vi "ProjetoB_59939_60461.vi"() -> ()   [LabVIEW 2024]
uses:
  <vilib>/Instr/_visa.llb/VISA Configure Serial Port (Instr).vi
  <vilib>/Analysis/NI_AALBase.lvlib
panel:
  in  "Help Button":bool
  out "Desvio Padrão Alto":bool
  in  "Limiar Desvio Padrão":dbl
  out "Desvio Padrão":dbl
  out "Frequência":dbl(graph)
  out "Array":dbl[](array[numeric])
  in  "Array - Numeric":dbl[](array[numeric])
  out "Sinal":u8(graph)
  in  "Ignição":bool
  in  "Modo\nAutomático":bool
  in  "Aumentar Frequência\n          Taxa Alta":bool
  in  "Aumentar Frequência\n         Taxa Baixa":bool
  in  "Reduzir \nFrequência":bool
  out "Sem onda há 10s":bool
  out "0.3 < Frequência < 0.6":bool
  in  "Iniciar/Parar \n  Aquisição":bool
  out "Frequência < 0.3":bool
  out "Frequência > 3":bool
  out "Deteção de Onda":bool
  in  "Limiar superior de Deteção":dbl=200.0
  out "Limiar inferior de Deteção":dbl=120.0
  out "Frequência":dbl
  in  "Taxa de Amostragem":u16(ring)=1 items=["25 S/s", "50 S/s", "100 S/s", "200 S/s"]
  in  "Gravar":bool
  out "Último Valor":dbl
  out "Error Out":errorcluster
  in  "stop":bool
  in  "Error In (no error)":errorcluster
  in  "Nome da Fonte VISA":refnum<visa-resource-name>="COM4"
  # "Monitorização de Plasma"
  # "Instrumentação Digital"
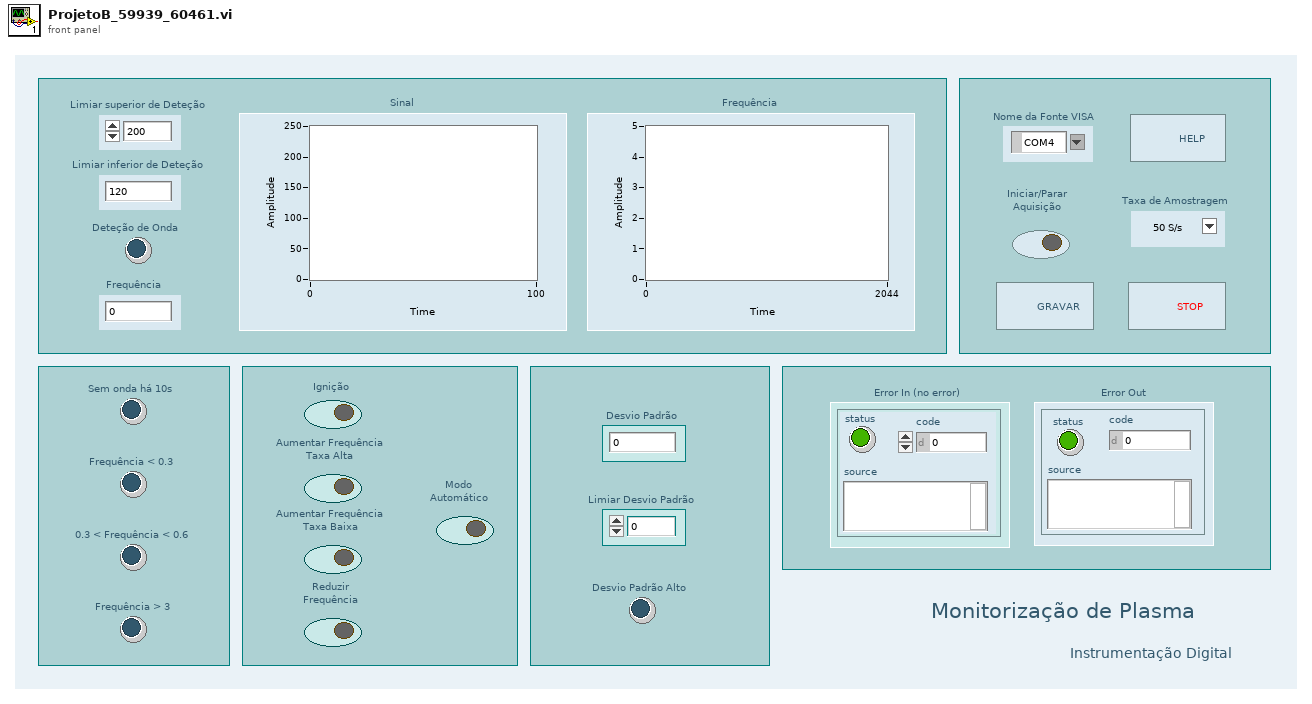
[diagram p1: front panel]
types:
  T1 = enum16{"open", "replace", "create", "open or create", "replace or create", "replace or create with confirmation"}
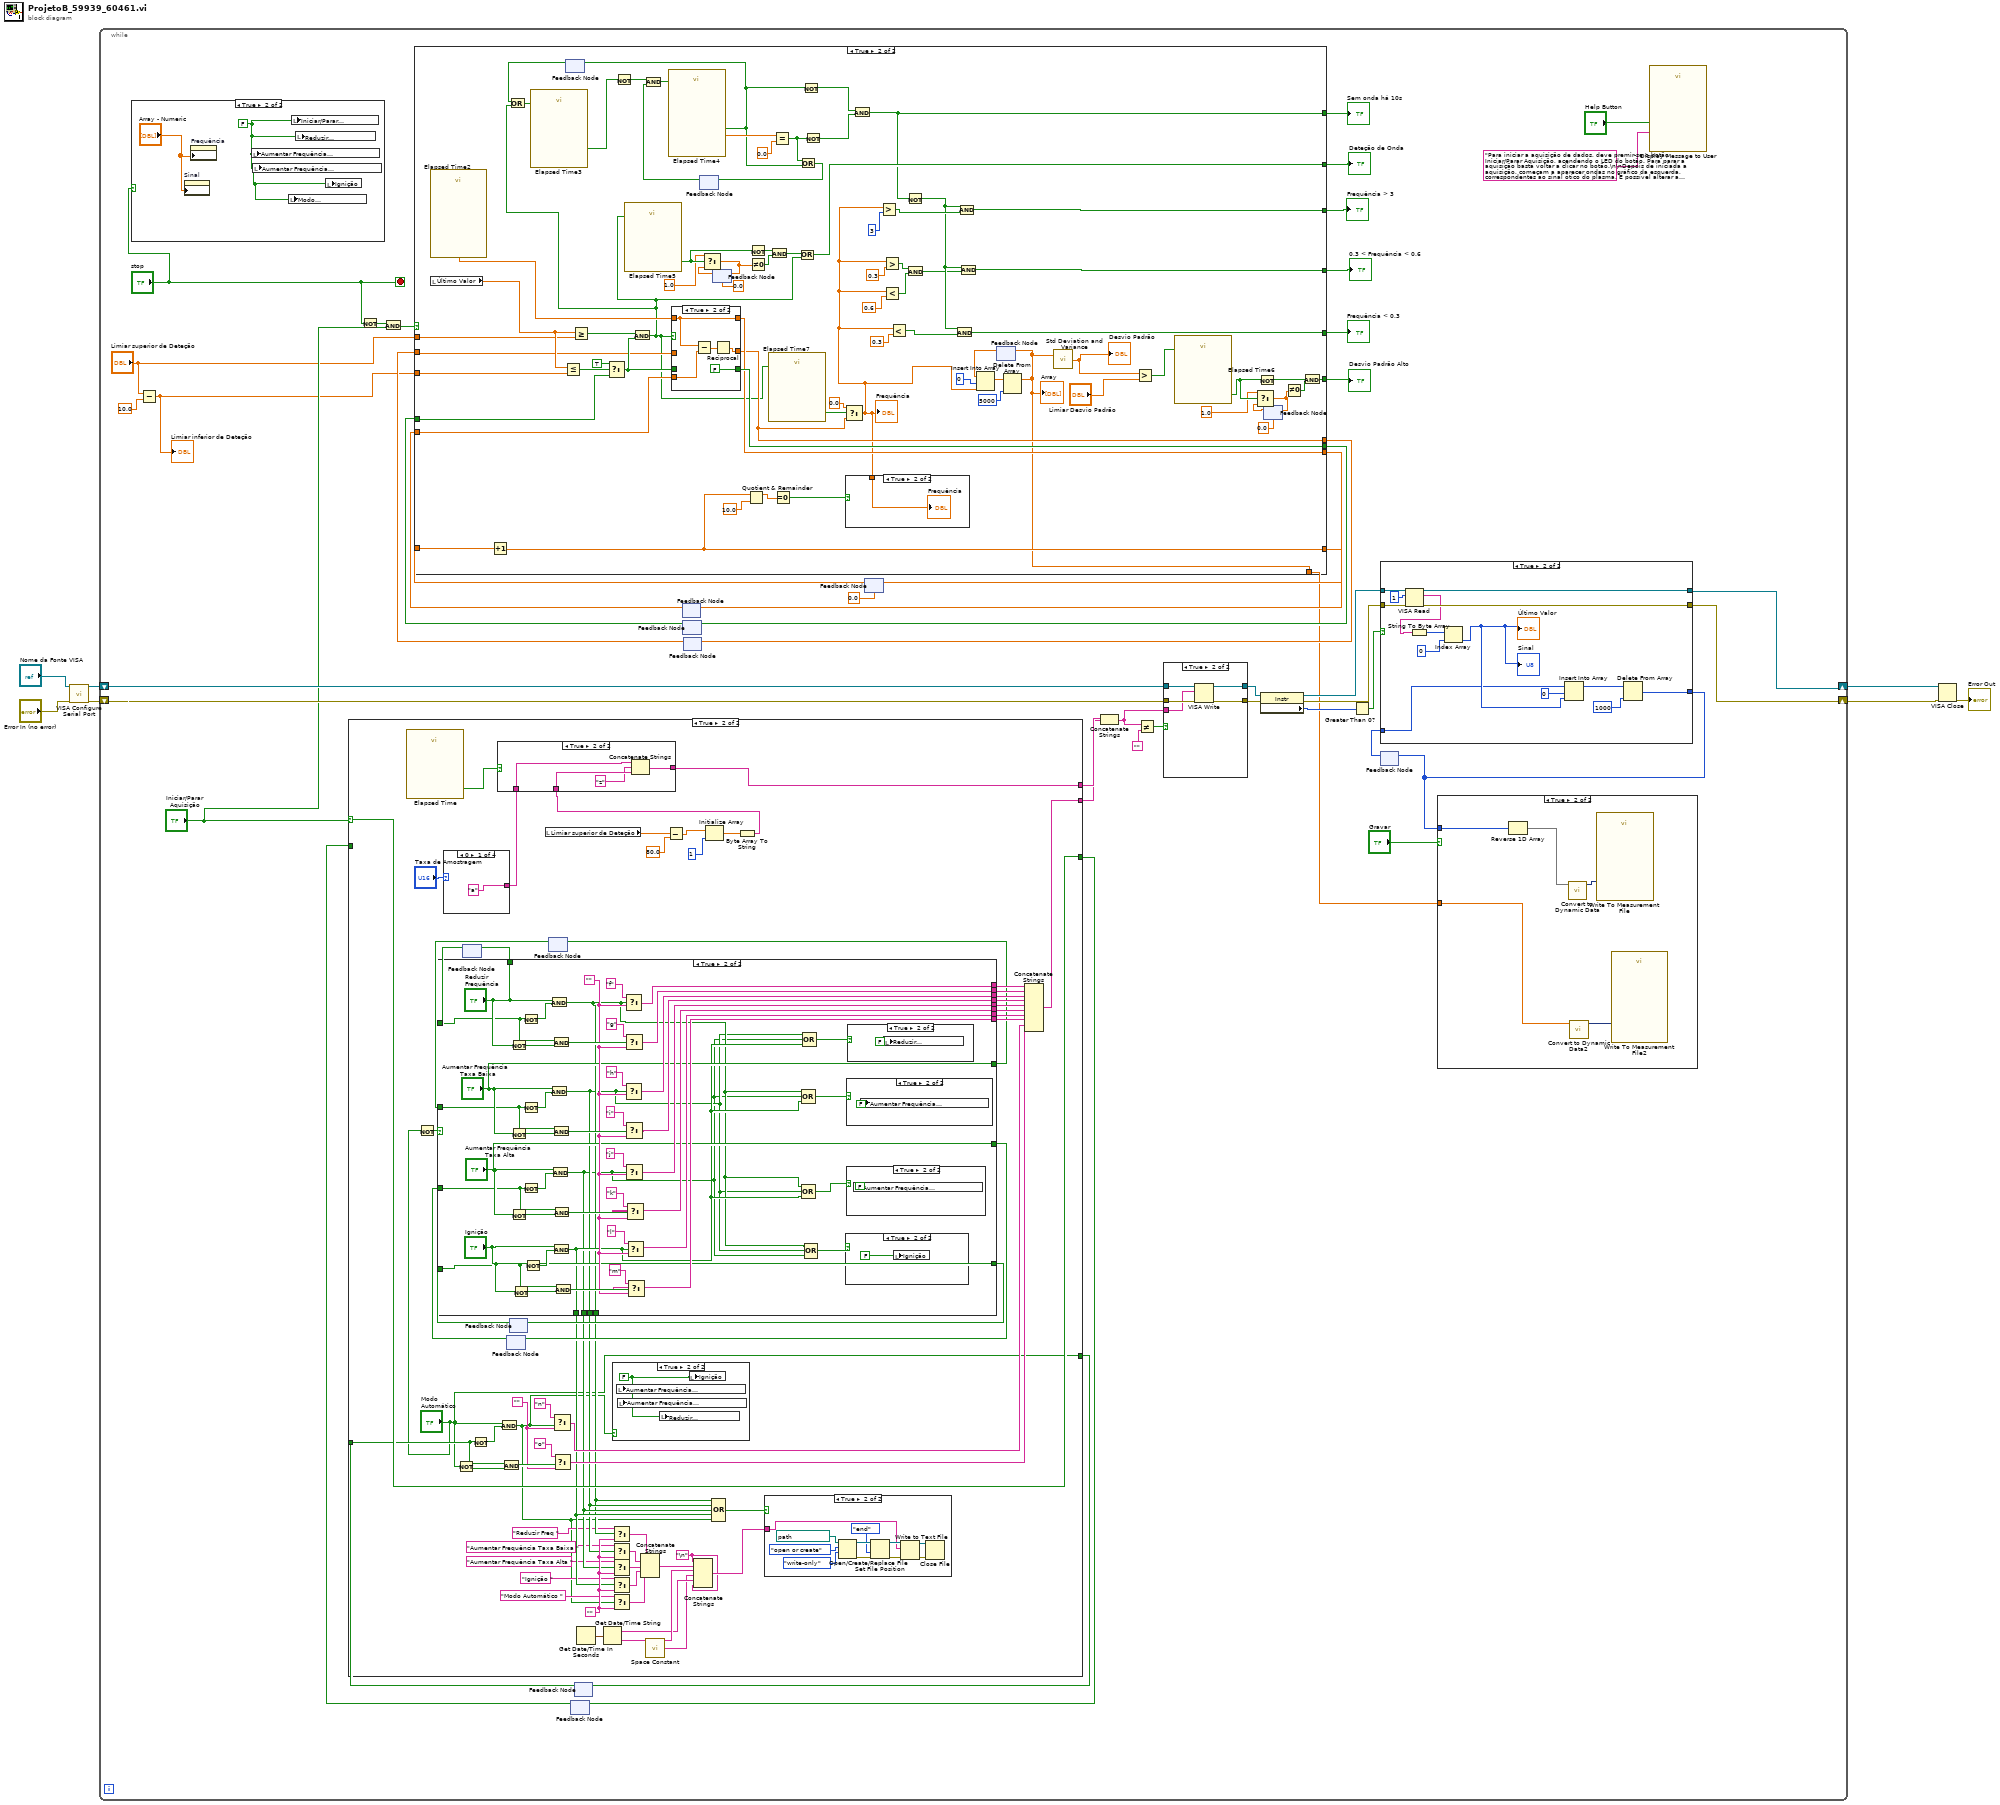
[diagram p0: block diagram]
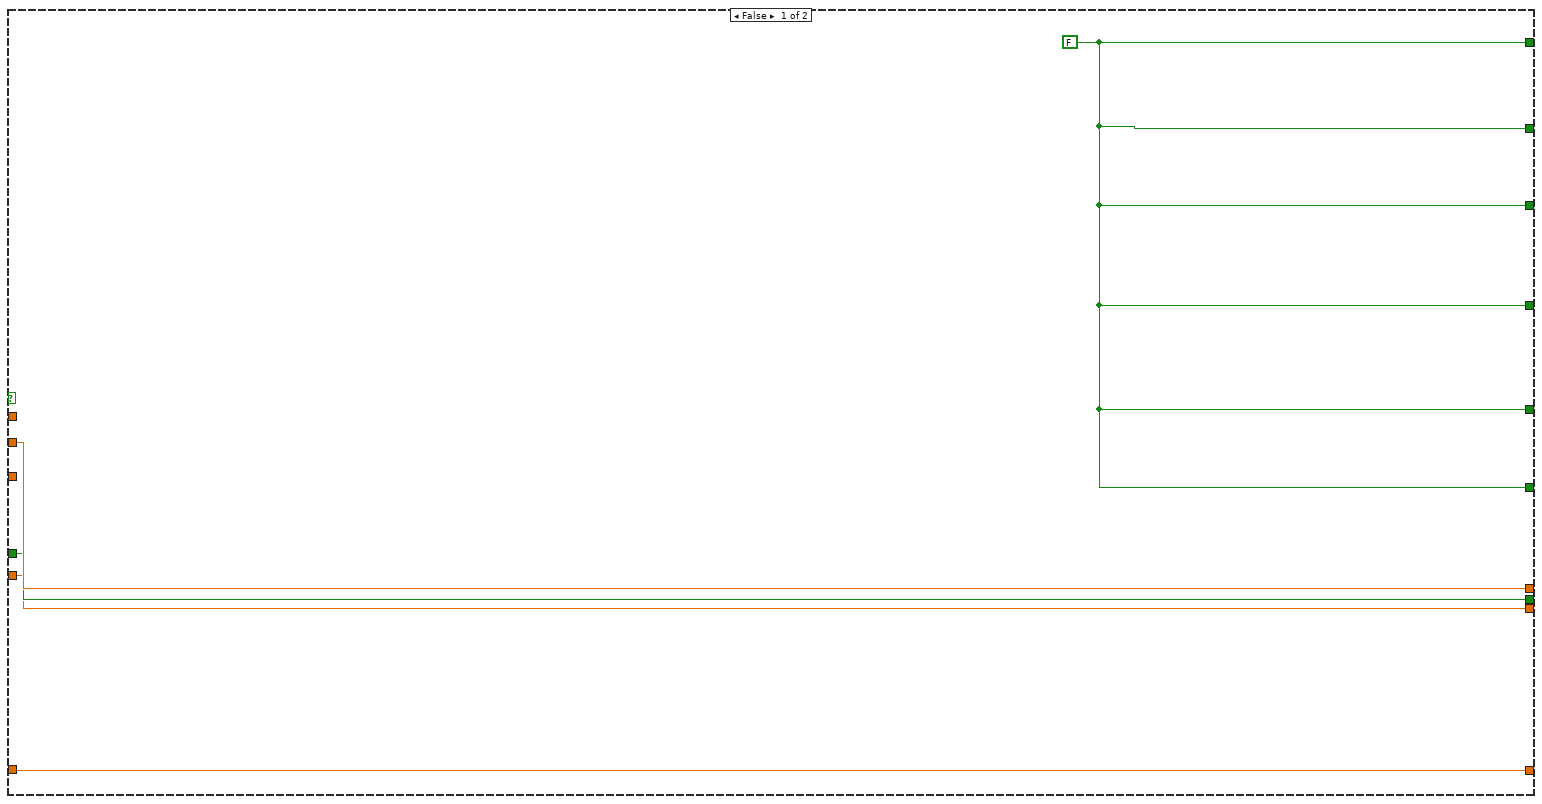
[diagram p3: hidden frame]
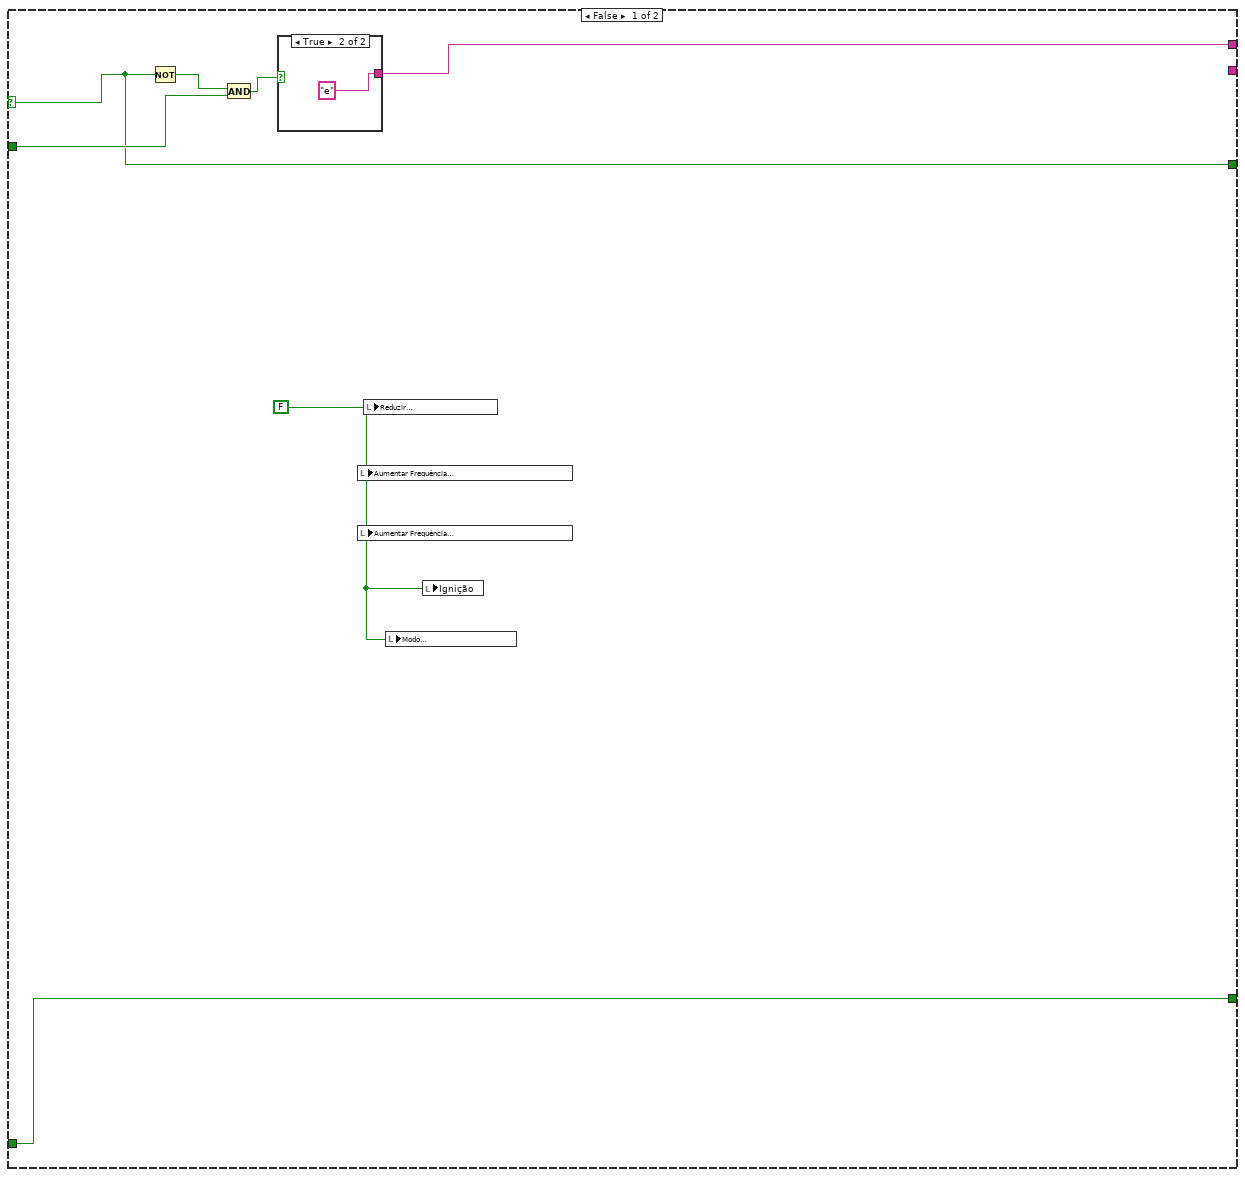
[diagram p6: hidden frame]
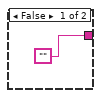
[diagram p7: hidden frame]
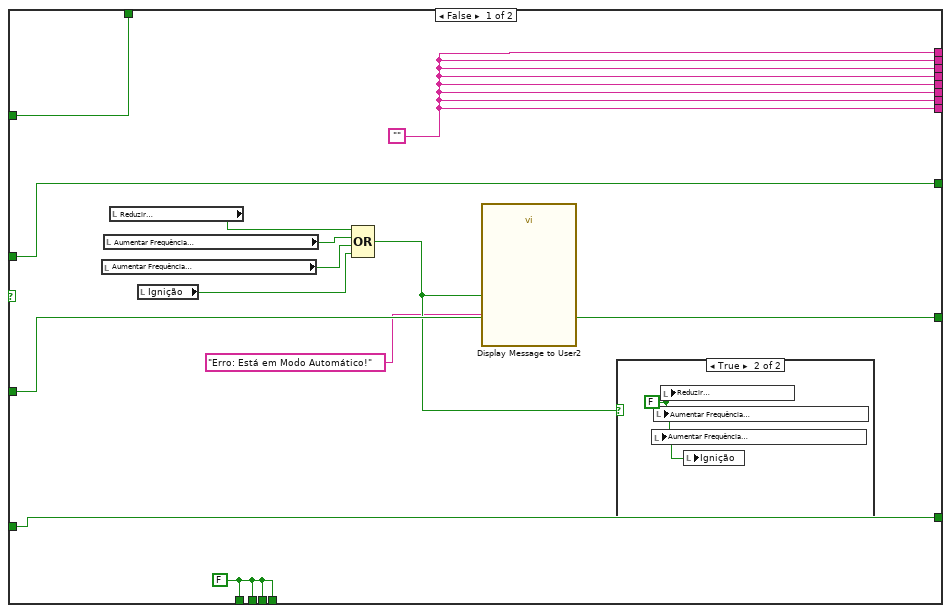
[diagram p10: hidden frame]
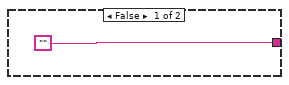
[diagram p16: hidden frame]
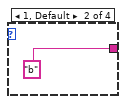
[diagram p17: hidden frame]
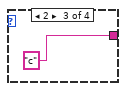
[diagram p18: hidden frame]
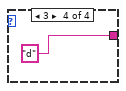
[diagram p19: hidden frame]
diagram:
  n1 = call-poly "VISA Configure Serial Port"("VISA resource name"="Nome da Fonte VISA", "error in (no error)"="Error In (no error)") -> ("VISA resource name out"=w5:refnum<visa-resource-name>, "error out"=w4:errorcluster)  [unwired: 12 in]
  n2 = while {
    shift-right: [w51] -> w3
    shift-left: w5 -> [w49]
    shift-right: [w50] -> w2
    shift-left: w4 -> [w48]
    stop <- "stop" stop-if-true
    n3 = case shown="True" "stop" {
      frame False {
      }
      frame True {
        w55 = FALSE
        n4 = property on="Sinal" class="WFChart (strict)"("History Data"="Array - Numeric") -> ()  [unwired: 2 in, 2 out]
        n5 = property on="Frequência" class="WFChart (strict)"("History Data"="Array - Numeric") -> ()  [unwired: 2 in, 2 out]
        n6 = local write "Aumentar Frequência\n         Taxa Baixa"(w55) -> ()
        n7 = local write "Aumentar Frequência\n          Taxa Alta"(w55) -> ()
        n8 = local write "Modo\nAutomático"(w55) -> ()
        n9 = local write "Iniciar/Parar \n  Aquisição"(w55) -> ()
        n10 = local write "Reduzir \nFrequência"(w55) -> ()
        n11 = local write "Ignição"(w55) -> ()
      }
    }
    n12 = Subtract(x="Limiar superior de Deteção", y=10.0) -> (x-y=w13:dbl)
    "Limiar inferior de Deteção" <- w13
    n13 = Not(x="stop") -> (.not. x?=w21:bool)
    n14 = And(x=w21, y="Iniciar/Parar \n  Aquisição") -> (x .and. y?=w23:bool)
    n15 = feedback #1() -> (w40:bool)  [unwired: 1 in]
    n16 = feedback #2() -> (w10:bool)  [unwired: 1 in]
    n17 = case shown="True" "Iniciar/Parar \n  Aquisição" {
      selector: "Iniciar/Parar \n  Aquisição" -> [w148 w214]
      tunnel: [w149 w215] -> w33
      tunnel: [w148 w214] -> w41
      tunnel: w40 -> [w151 _]
      tunnel: [_ w211] -> w31
      tunnel: w10 -> [w147 w157]
      tunnel: [w147 "Modo\nAutomático"] -> w11
      frame False {
        w146 = FALSE
        n18 = Not(x=w148) -> (.not. x?=w152:bool)
        n19 = And(x=w152, y=w151) -> (x .and. y?=w150:bool)
        n20 = case shown="True" w150 {
          tunnel: ["" "e" ("Write 2")] -> w149
          frame False {
          }
          frame True {
          }
        }
        n21 = local write "Aumentar Frequência\n         Taxa Baixa"(w146) -> ()
        n22 = local write "Aumentar Frequência\n          Taxa Alta"(w146) -> ()
        n23 = local write "Reduzir \nFrequência"(w146) -> ()
        n24 = local write "Modo\nAutomático"(w146) -> ()
        n25 = local write "Ignição"(w146) -> ()
      }
      frame True {
        w167 = ""
        w175 = "\n"
        w201 = ""
        n26 = call "Elapsed Time"() -> ("Time has Elapsed"=w217:bool)  [unwired: 12 in, 7 out]
        n27 = Not(x="Modo\nAutomático") -> (.not. x?=w198:bool)
        n28 = case shown="0" "Taxa de Amostragem" {
          tunnel: ["a" ("Write 2") "b" ("Write 2") "c" ("Write 2") "d" ("Write 2")] -> w216
          frame 0 {
          }
          frame 1, Default {
          }
          frame 2 {
          }
          frame 3 {
          }
        }
        n29 = Not(x="Modo\nAutomático") -> (.not. x?=w204:bool)
        n30 = feedback #3() -> (w189:bool)  [unwired: 1 in]
        n31 = Not(x=w157) -> (.not. x?=w202:bool)
        n32 = And(x="Modo\nAutomático", y=w202) -> (x .and. y?=w155:bool)
        n33 = And(x=w157, y=w204) -> (x .and. y?=w203:bool)
        n34 = feedback #4() -> (w191:bool)  [unwired: 1 in]
        n35 = feedback #5() -> (w193:bool)  [unwired: 1 in]
        n36 = local read "Limiar superior de Deteção"() -> (w183:dbl)
        n37 = feedback #6() -> (w187:bool)  [unwired: 1 in]
        n38 = case shown="True" w198 {
          tunnel: [w241 w282] -> w213
          tunnel: [w241 w281] -> w212
          tunnel: [w241 w275] -> w210
          tunnel: [w241 w274] -> w209
          tunnel: [w241 w268] -> w208
          tunnel: [w241 w267] -> w207
          tunnel: [w241 w260] -> w206
          tunnel: [w241 w259] -> w205
          tunnel: [w239 "Ignição"] -> w194
          tunnel: w193 -> [w239 w257]
          tunnel: [w240 "Aumentar Frequência\n          Taxa Alta"] -> w192
          tunnel: w191 -> [w240 w255]
          tunnel: [w237 "Aumentar Frequência\n         Taxa Baixa"] -> w188
          tunnel: [w238 "Reduzir \nFrequência"] -> w190
          tunnel: w189 -> [w238 w252]
          tunnel: w187 -> [w237 w251]
          tunnel: [w236 w247] -> w165
          tunnel: [w236 w243] -> w164
          tunnel: [w236 w244] -> w163
          tunnel: [w236 w245] -> w162
          frame False {
            w236 = FALSE
            w241 = ""
            n39 = local read "Aumentar Frequência\n          Taxa Alta"() -> (w233:bool)
            n40 = local read "Aumentar Frequência\n         Taxa Baixa"() -> (w234:bool)
            n41 = local read "Reduzir \nFrequência"() -> (w235:bool)
            n42 = local read "Ignição"() -> (w232:bool)
            n43 = Compound Arithmetic op=OR(w235, w234, w233, w232) -> (w231:bool)
            n44 = call "Display Message to User2"("Enable"=w231, "Message"="Erro: Está em Modo Automático!") -> ()  [unwired: 8 in, 2 out]
            n45 = case shown="True" w231 {
              frame False {
              }
              frame True {
                w242 = FALSE
                n46 = local write "Aumentar Frequência\n          Taxa Alta"(w242) -> ()
                n47 = local write "Aumentar Frequência\n         Taxa Baixa"(w242) -> ()
                n48 = local write "Reduzir \nFrequência"(w242) -> ()
                n49 = local write "Ignição"(w242) -> ()
              }
            }
          }
          frame True {
            w261 = ""
            n50 = Not(x="Reduzir \nFrequência") -> (.not. x?=w283:bool)
            n51 = Not(x="Aumentar Frequência\n         Taxa Baixa") -> (.not. x?=w276:bool)
            n52 = Not(x="Aumentar Frequência\n          Taxa Alta") -> (.not. x?=w269:bool)
            n53 = Not(x="Ignição") -> (.not. x?=w262:bool)
            n54 = Not(x=w252) -> (.not. x?=w287:bool)
            n55 = Not(x=w251) -> (.not. x?=w280:bool)
            n56 = Not(x=w255) -> (.not. x?=w273:bool)
            n57 = Not(x=w257) -> (.not. x?=w266:bool)
            n58 = And(x="Reduzir \nFrequência", y=w287) -> (x .and. y?=w245:bool)
            n59 = And(x="Aumentar Frequência\n         Taxa Baixa", y=w280) -> (x .and. y?=w244:bool)
            n60 = And(x="Aumentar Frequência\n          Taxa Alta", y=w273) -> (x .and. y?=w243:bool)
            n61 = And(x=w252, y=w283) -> (x .and. y?=w284:bool)
            n62 = And(x=w251, y=w276) -> (x .and. y?=w277:bool)
            n63 = And(x="Ignição", y=w266) -> (x .and. y?=w247:bool)
            n64 = And(x=w255, y=w269) -> (x .and. y?=w270:bool)
            n65 = And(x=w257, y=w262) -> (x .and. y?=w263:bool)
            n66 = Select(t="f", s=w245, f=w261) -> (s? t:f=w282:string)
            n67 = Select(t="h", s=w244, f=w261) -> (s? t:f=w275:string)
            n68 = Select(t="g", s=w284, f=w261) -> (s? t:f=w281:string)
            n69 = Select(t="i", s=w277, f=w261) -> (s? t:f=w274:string)
            n70 = Select(t="j", s=w243, f=w261) -> (s? t:f=w268:string)
            n71 = Select(t="k", s=w270, f=w261) -> (s? t:f=w267:string)
            n72 = Select(t="l", s=w247, f=w261) -> (s? t:f=w260:string)
            n73 = Select(t="m", s=w263, f=w261) -> (s? t:f=w259:string)
            n74 = Compound Arithmetic op=OR(w245, w243, w247) -> (w248:bool)
            n75 = Compound Arithmetic op=OR(w245, w244, w247) -> (w249:bool)
            n76 = Compound Arithmetic op=OR(w244, w243, w247) -> (w250:bool)
            n77 = Compound Arithmetic op=OR(w245, w244, w243) -> (w246:bool)
            n78 = case shown="True" w246 {
              frame False {
              }
              frame True {
                n79 = local write "Ignição"(FALSE) -> ()
              }
            }
            n80 = case shown="True" w248 {
              frame False {
              }
              frame True {
                n81 = local write "Aumentar Frequência\n         Taxa Baixa"(FALSE) -> ()
              }
            }
            n82 = case shown="True" w249 {
              frame False {
              }
              frame True {
                n83 = local write "Aumentar Frequência\n          Taxa Alta"(FALSE) -> ()
              }
            }
            n84 = case shown="True" w250 {
              frame False {
              }
              frame True {
                n85 = local write "Reduzir \nFrequência"(FALSE) -> ()
              }
            }
          }
        }
        n86 = feedback-in #3(w190) -> ()
        n87 = feedback-in #4(w192) -> ()
        n88 = feedback-in #5(w194) -> ()
        n89 = feedback-in #6(w188) -> ()
        n90 = Select(t="n", s=w155, f=w201) -> (s? t:f=w197:string)
        n91 = Select(t="o", s=w203, f=w201) -> (s? t:f=w196:string)
        n92 = Get Date/Time In Seconds() -> (seconds since 1Jan1904=w179:timestamp)
        n93 = Get Date/Time String(seconds (now)=w179) -> (date string=w177:string, time string=w178:string)  [unwired: 2 in]
        n94 = case shown="True" w155 {
          frame False {
          }
          frame True {
            w218 = FALSE
            n95 = local write "Aumentar Frequência\n          Taxa Alta"(w218) -> ()
            n96 = local write "Aumentar Frequência\n         Taxa Baixa"(w218) -> ()
            n97 = local write "Reduzir \nFrequência"(w218) -> ()
            n98 = local write "Ignição"(w218) -> ()
          }
        }
        n99 = Select(t="Reduzir Freq ", s=w162, f=w167) -> (s? t:f=w168:string)
        n100 = Select(t="Aumentar Frequência Taxa Baixa ", s=w163, f=w167) -> (s? t:f=w169:string)
        n101 = Select(t="Aumentar Frequência Taxa Alta ", s=w164, f=w167) -> (s? t:f=w172:string)
        n102 = Select(t="Ignição ", s=w165, f=w167) -> (s? t:f=w171:string)
        n103 = Select(t="Modo Automático ", s=w155, f=w167) -> (s? t:f=w170:string)
        n104 = Concatenate Strings(w168, w169, w172, w171, w170) -> (w173:string)
        n105 = call <vilib>:"Space Constant.vi"() -> ("String"=w176:string)
        n106 = Subtract(x=w183, y=80.0) -> (x-y=w182:dbl)
        n107 = Concatenate Strings(w175, w173, w178, w176, w177, w175) -> (w180:string)
        n108 = Initialize Array(w182, 1) -> (w185:dbl[])
        n109 = Compound Arithmetic op=OR(w162, w163, w164, w165, w155) -> (w174:bool)
        n110 = Byte Array To String(unsigned byte array=w185) -> (string=w181:string)
        n111 = case shown="True" w217 {
          tunnel: w216 -> [_ w296]
          tunnel: ["" w295] -> w215
          tunnel: w181 -> [_ w294]
          frame False {
          }
          frame True {
            n112 = Concatenate Strings(w296, "z", w294) -> (w295:string)
          }
        }
        n113 = case shown="True" w174 {
          tunnel: w180 -> [_ w220]
          frame False {
          }
          frame True {
            n114 = Open/Create/Replace File(file path (use dialog)=path "C:/Users/ruira/OneDrive/Ambiente de Trabalho/4ºano/2ºsemestre/ID/ProjetoB-59939-60461/DataLabView/Log_0.txt", operation (0:open)=T1."open or create", access (0:read/write)=enum16{"read/write", "read-only", "write-only"}."write-only") -> (refnum out=w227:refnum<file>, error out=w224:errorcluster)  [unwired: 3 in, 1 out]
            n115 = Set File Position(refnum=w227, from (0:start)=enum16{"start", "end", "current"}."end", error in=w224) -> (refnum out=w225:refnum<file>, error out=w223:errorcluster)  [unwired: 1 in]
            n116 = Write to Text File(file (use dialog)=w225, text=w220, error in=w223) -> (refnum out=w221:refnum<file>, error out=w222:errorcluster)  [unwired: 1 in, 1 out]
            n117 = Close File(refnum=w221, error in=w222) -> ()  [unwired: 2 out]
          }
        }
        n118 = Concatenate Strings(w213, w212, w210, w209, w208, w207, w206, w205, w197, w196) -> (w211:string)
      }
    }
    n119 = feedback-in #1(w41) -> ()
    n120 = feedback-in #2(w11) -> ()
    n121 = feedback #7() -> (w35:dbl)  [unwired: 1 in]
    n122 = feedback #8() -> (w38:bool)  [unwired: 1 in]
    n123 = feedback #9() -> (w37:dbl)  [unwired: 1 in]
    n124 = feedback #10(0.0) -> (w17:dbl)
    n125 = case shown="True" w23 {
      tunnel: [w60 w125] -> w39
      tunnel: w38 -> [w60 w124]
      tunnel: w37 -> [w61 w122]
      tunnel: [w61 w72] -> w36
      tunnel: w35 -> [w59 w121]
      tunnel: [w59 w123] -> w34
      tunnel: [w58 w98] -> w28
      tunnel: [w58 w102] -> w27
      tunnel: [w58 w101] -> w26
      tunnel: [w58 w100] -> w25
      tunnel: [w58 w99] -> w24
      tunnel: [w58 w85] -> w19
      tunnel: [w57 w66] -> w18
      tunnel: w17 -> [w57 w71]
      tunnel: "Limiar superior de Deteção" -> [_ w65]
      tunnel: w13 -> [_ w64]
      tunnel: [_ w62] -> w12
      frame False {
        w58 = FALSE
      }
      frame True {
        n126 = call "Elapsed Time2"() -> ("Elapsed Time (s)"=w132:dbl)  [unwired: 12 in, 7 out]
        n127 = local read "Último Valor"() -> (w133:dbl)
        n128 = Increment(x=w71) -> (x+1=w66:dbl)
        n129 = Less Or Equal?(x=w133, y=w64) -> (x <= y?=w135:bool)
        n130 = feedback #11() -> (w108:bool)  [unwired: 1 in]
        n131 = Greater Or Equal?(x=w133, y=w65) -> (x >= y?=w120:bool)
        n132 = Select(t=TRUE, s=w135, f=w124) -> (s? t:f=w136:bool)
        n133 = And(x=w120, y=w136) -> (x .and. y?=w63:bool)
        n134 = Or(x=w108, y=w63) -> (x .or. y?=w107:bool)
        n135 = call "Elapsed Time3"("Reset"=w107) -> ("Time has Elapsed"=w109:bool)  [unwired: 11 in, 7 out]
        n136 = Not(x=w109) -> (.not. x?=w118:bool)
        n137 = call "Elapsed Time5"("Reset"=w63) -> ("Time has Elapsed"=w79:bool)  [unwired: 11 in, 7 out]
        n138 = case shown="True" w63 {
          tunnel: [w140 FALSE] -> w125
          tunnel: w136 -> [w140 _]
          tunnel: w132 -> [_ w144]
          tunnel: [w139 w144] -> w123
          tunnel: w121 -> [w139 w143]
          tunnel: [w138 w141] -> w72
          tunnel: w122 -> [w138 _]
          frame False {
          }
          frame True {
            n139 = Subtract(x=w144, y=w143) -> (x-y=w142:dbl)
            n140 = Reciprocal(x=w142) -> (1/x=w141:dbl)
          }
        }
        n141 = feedback #12() -> (w115:bool)  [unwired: 1 in]
        n142 = And(x=w118, y=w115) -> (x .and. y?=w119:bool)
        n143 = call "Elapsed Time4"("Reset"=w119) -> ("Elapsed Time (s)"=w114:dbl, "Time has Elapsed"=w103:bool)  [unwired: 11 in, 6 out]
        n144 = feedback-in #11(w103) -> ()
        n145 = feedback #13(0.0) -> (w82:dbl)
        n146 = Select(t=1.0, s=w79, f=w82) -> (s? t:f=w80:dbl)
        n147 = feedback-in #13(w80) -> ()
        n148 = Quotient & Remainder(x=w66, y=10.0) -> (x-y*floor(x/y)=w70:dbl)  [unwired: 1 out]
        n149 = Not(x=w79) -> (.not. x?=w76:bool)
        n150 = Not Equal To 0?(x=w80) -> (x != 0?=w77:bool)
        n151 = call "Elapsed Time7"("Reset"=w63) -> ("Time has Elapsed"=w74:bool)  [unwired: 11 in, 7 out]
        n152 = And(x=w76, y=w77) -> (x .and. y?=w78:bool)
        n153 = Equal?(x=w114, y=0.0) -> (x = y?=w104:bool)
        n154 = Equal To 0?(x=w70) -> (x = 0?=w69:bool)
        n155 = Or(x=w78, y=w63) -> (x .or. y?=w99:bool)
        n156 = Or(x=w104, y=w103) -> (x .or. y?=w116:bool)
        n157 = feedback-in #12(w116) -> ()
        n158 = Not(x=w103) -> (.not. x?=w106:bool)
        n159 = Not(x=w104) -> (.not. x?=w105:bool)
        n160 = Select(t=0.0, s=w74, f=w72) -> (s? t:f=w68:dbl)
        "Frequência" <- w68
        n161 = case shown="True" w69 {
          tunnel: w68 -> [_ w137]
          frame False {
          }
          frame True {
            "Frequência" <- w137
          }
        }
        n162 = And(x=w106, y=w105) -> (x .and. y?=w98:bool)
        n163 = Greater?(x=w68, y=3) -> (0:w113:bool)
        n164 = Greater?(x=w68, y=0.3) -> (0:w130:bool)
        n165 = Less?(x=w68, y=0.6) -> (x < y?=w129:bool)
        n166 = Less?(x=w68, y=0.3) -> (x < y?=w110:bool)
        n167 = Not(x=w98) -> (.not. x?=w112:bool)
        n168 = And(x=w130, y=w129) -> (x .and. y?=w111:bool)
        n169 = And(x=w112, y=w110) -> (x .and. y?=w100:bool)
        n170 = And(x=w112, y=w113) -> (x .and. y?=w102:bool)
        n171 = And(x=w112, y=w111) -> (x .and. y?=w101:bool)
        n172 = feedback #14() -> (w94:dbl[])  [unwired: 1 in]
        n173 = Insert Into Array(array=w94, index=0, new element=w68) -> (w95:dbl[])
        n174 = Delete From Array(array=w95, index=5000) -> (array with subset deleted=w62:dbl[])  [unwired: 1 in, 1 out]
        "Array" <- w62
        n175 = feedback-in #14(w62) -> ()
        n176 = call <vilib>:"Std Deviation and Variance.vi"("X"=w62) -> ("standard deviation"=w93:dbl)  [unwired: 1 in, 2 out]
        "Desvio Padrão" <- w93
        n177 = Greater?(x=w93, y="Limiar Desvio Padrão") -> (0:w91:bool)
        n178 = call "Elapsed Time6"("Reset"=w91) -> ("Time has Elapsed"=w90:bool)  [unwired: 11 in, 7 out]
        n179 = Not(x=w90) -> (.not. x?=w83:bool)
        n180 = feedback #15(0.0) -> (w88:dbl)
        n181 = Select(t=1.0, s=w90, f=w88) -> (s? t:f=w86:dbl)
        n182 = feedback-in #15(w86) -> ()
        n183 = Not Equal To 0?(x=w86) -> (x != 0?=w84:bool)
        n184 = And(x=w83, y=w84) -> (x .and. y?=w85:bool)
      }
    }
    "Sem onda há 10s" <- w28
    "Frequência > 3" <- w27
    "0.3 < Frequência < 0.6" <- w26
    "Frequência < 0.3" <- w25
    "Deteção de Onda" <- w24
    "Desvio Padrão Alto" <- w19
    n185 = feedback-in #7(w34) -> ()
    n186 = feedback-in #8(w39) -> ()
    n187 = feedback-in #9(w36) -> ()
    n188 = feedback-in #10(w18) -> ()
    n189 = Concatenate Strings(w33, w31) -> (w32:string)
    n190 = Not Equal?(x=w32, y="") -> (x != y?=w45:bool)
    n191 = case shown="True" w45 {
      tunnel: w49 -> [w307 w310]
      tunnel: w48 -> [w306 w309]
      tunnel: [w307 w312] -> w47
      tunnel: [w306 w311] -> w46
      tunnel: w32 -> [_ w308]
      frame False {
      }
      frame True {
        n192 = VISA Write(VISA resource name=w310, write buffer=w308, error in (no error)=w309) -> (VISA resource name out=w312:refnum<visa-resource-name>, error out=w311:errorcluster)  [unwired: 1 out]
      }
    }
    n193 = property class="Instr"(reference=w47, error in=w46) -> (reference out=w53:refnum<visa-resource-name>, error out=w52:errorcluster, "Serial Settings:Number of Bytes at Serial Port"=w54:u32)
    n194 = Greater Than 0?(x=w54) -> (x > 0?=w42:bool)
    n195 = feedback #16() -> (w30:u8[])  [unwired: 1 in]
    n196 = case shown="True" w42 {
      tunnel: w53 -> [w315 w328]
      tunnel: w52 -> [w314 w329]
      tunnel: [w315 w326] -> w51
      tunnel: [w314 w325] -> w50
      tunnel: [w313 w317] -> w29
      tunnel: w30 -> [w313 w316]
      frame False {
      }
      frame True {
        n197 = VISA Read(VISA resource name=w328, byte count=u32 1, error in (no error)=w329) -> (VISA resource name out=w326:refnum<visa-resource-name>, read buffer=w323:string, error out=w325:errorcluster)  [unwired: 1 out]
        n198 = String To Byte Array(string=w323) -> (unsigned byte array=w324:u8[])
        n199 = Index Array(array=w324, index=0) -> (element=w318:u8)
        "Último Valor" <- w318
        "Sinal" <- w318
        n200 = Insert Into Array(array=w316, index=0, new element=w318) -> (w319:u8[])
        n201 = Delete From Array(array=w319, index=1000) -> (array with subset deleted=w317:u8[])  [unwired: 1 in, 1 out]
      }
    }
    n202 = feedback-in #16(w29) -> ()
    n203 = case shown="True" "Gravar" {
      tunnel: w29 -> [_ w305]
      tunnel: w12 -> [_ w301]
      frame False {
      }
      frame True {
        n204 = Reverse 1D Array(array=w305) -> (reversed array=w302:u8[])
        n205 = call "Convert to Dynamic Data"("Array"=w302) -> ("Dynamic Data Type"=w304:dynamicdata)  [unwired: 3 in]
        n206 = call "Convert to Dynamic Data2"("Array"=w301) -> ("Dynamic Data Type"=w303:dynamicdata)  [unwired: 3 in]
        n207 = call "Write To Measurement File"("Signals"=w304) -> ()  [unwired: 16 in, 3 out]
        n208 = call "Write To Measurement File2"("Signals"=w303) -> ()  [unwired: 16 in, 3 out]
      }
    }
    n209 = call "Display Message to User"("Enable"="Help Button", "Message"="Para iniciar a aquisição de dados, deve premir-se o botão Iniciar/Parar Aquisição, acendendo o LED do botão. Para parar a aquisição basta voltar a clicar no botão.\n\nDepois de iniciada a aquisição, começam a aparecer ondas no gráfico da esquerda, correspondentes ao sinal ótico do plasma. É possível alterar a taxa de amostragem no menu drop down, bem como gravar os dados recebidos (1000 últimos valores de sinal e 5000 frequências) no botão correspondente.\n\nO utilizador deve ajustar o limiar superior de deteção no controlador correspondente, sendo o limiar inferior alterado automaticamente, de modo a que a onda principal seja a única a ultrapassar o limiar superior, e que esta intercete também o limiar inferior. Por cada onda que é detetada, o LED de Deteção de Onda pisca. A frequência do sinal pode ser observada no mostrador Frequência. O gráfico da direita mostra a evolução da frequência ao longo do tempo.\n\nSe a frequência for superior a 3Hz, o LED correspondente acende, e o mesmo para se for entre 0.3Hz e 0.6Hz, e se for menor que 0.3Hz. Se não for detetada nenhuma onda num período de 10 segundos, o LED correspondente é ativado, permanecendo ativado durante 5 segundos, independentemente de virem a ser detetadas ondas nesse período. Após o LED apagar, se voltarem a passar 10 segundos sem deteção de ondas, repete-se o processo.\n\nSe houver grandes variações de frequência, o LED de Desvio Padrão Alto é ativado. O limiar para o desvio padrão pode ser ajustado pelo utilizador no respetivo controlador.\n\nPara atuar sobre a informação dada pelos LEDs, há 4 botões de ação correspondentes: Ignição, para quando não são detetadas ondas há mais de 10s; Aumentar a frequência a uma taxa alta, para quando esta é inferior a 0.3Hz; Aumentar a frequência a uma taxa baixa, para quando esta está entre 0.3Hz e 0.6Hz; Reduzir frequência, para quando esta é superior a 3Hz. Ao clicar nestes botões, os LEDs físicos acendem, correspondendo às ações que devem ser efetuadas.\n\nAo clicar no botão de modo automático, os LEDs físicos passam a ser controlados automaticamente, deixando de ser necessário clicar nos botões de ação. Por exemplo, se a frequência for maior que 3Hz, o LED de redução de frequência é ativado automaticamente.\n\nQuando se clica num botão, a informação sobre a data, hora, e que botão foi premido é guardada num ficheiro de texto. Não se deve clicar em botões de ação enquanto se está em modo automático. Caso se tente fazer isto, irá aparecer um pop-up com uma mensagem de erro.\n\nO controlador Nome da Fonte VISA determina o port pelo qual os dados devem ser recebidos. Mensagens de erro relativas a esta fonte podem ser visualizadas nos mostradores Error In e Error Out.\n\nPara parar o programa, deve-se clicar no botão Stop.") -> ()  [unwired: 8 in, 2 out]
  }
  n210 = VISA Close(VISA resource name=w3, error in (no error)=w2) -> (error out=→"Error Out":errorcluster)
